vi "Performance Test 1.vi"() -> ()   [LabVIEW 2015, in "ByRef Variant Repository.lvlib"]
uses:
  ByRef Variant Repository.lvlib
  <vilib>/Analysis/1siggen.llb/Riffle Array (I32).vi
  <userlib>/_OpenG.lib/array/array.llb/Reorder 1D Array2 (String)__ogtk.vi
  <userlib>/_OpenG.lib/array/array.llb/Reorder 1D Array2 (SGL)__ogtk.vi
  <vilib>/Analysis/NI_AALBase.lvlib
panel:
  out "Data OK":bool
  out "Read Time [s]":dbl
  out "Write Time [s]":dbl
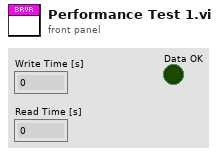
[diagram p1: front panel]
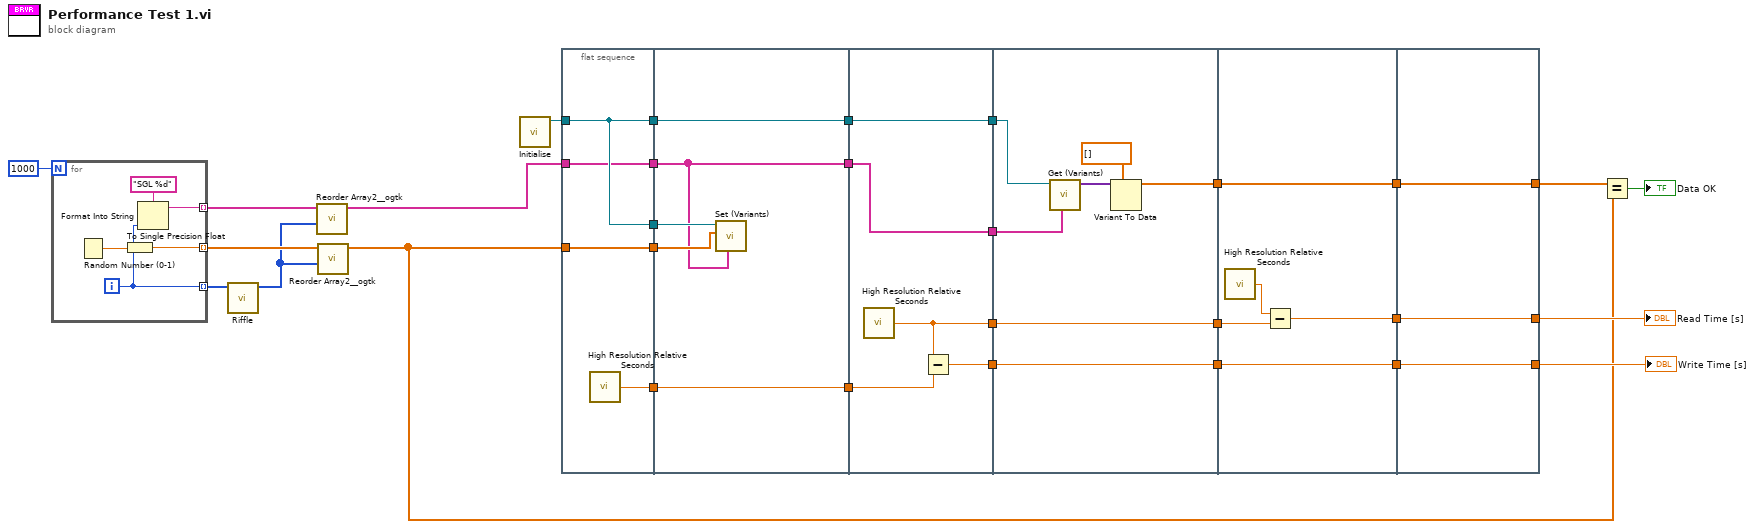
[diagram p0: block diagram]
diagram:
  n1 = for {
    N: 1000 -> [_]
    tunnel: [w34] -> w21 mode=indexing
    tunnel: [w32] -> w23 mode=indexing
    tunnel: [w31] -> w25 mode=indexing
    i -> [w31]
    n2 = Random Number (0-1)() -> (number: 0 to 1=w35:dbl)
    n3 = To Single Precision Float(number=w35) -> (single precision float=w34:sgl)
    n4 = Format Into String(format string="SGL %d", w31) -> (resulting string=w32:string)  [unwired: 2 in, 1 out]
  }
  n5 = call-poly <vilib>:"Riffle.vi"("X"=w25) -> ("Riffled {X}"=w20:i32[])  [unwired: 8 in, 2 out]
  n6 = call-poly <userlib>:"Reorder Array2__ogtk.vi"("indices"=w20, "array"=w23) -> ("reordered array"=w24:string[])  [unwired: 9 in]
  n7 = call-poly <userlib>:"Reorder Array2__ogtk.vi"("indices"=w20, "array"=w21) -> ("reordered array"=w22:sgl[])  [unwired: 9 in]
  n8 = call "Initialise.vi"() -> ("ByRef Variant Repsitory out"=w1:refnum<data-value>)  [unwired: 9 in, 1 out]
  n9 = flat-sequence {
    tunnel: w22 -> [w39]
    tunnel: w1 -> [w38]
    tunnel: [w38] -> w19
    tunnel: [w39] -> w18
    tunnel: [w38] -> w17
    tunnel: [w37] -> w16
    tunnel: w24 -> [w37]
    tunnel: [w36] -> w15
    tunnel: w19 -> [w42]
    tunnel: w18 -> [w41]
    tunnel: [w44] -> w14
    tunnel: w17 -> [w44]
    tunnel: [w40] -> w13
    tunnel: w16 -> [w40]
    tunnel: [w43] -> w12
    tunnel: w15 -> [w43]
    tunnel: [w49] -> w11
    tunnel: w14 -> [w49]
    tunnel: [w48] -> w10
    tunnel: w13 -> [w48]
    tunnel: w12 -> [w47]
    tunnel: [w46] -> w9
    tunnel: [w45] -> w8
    tunnel: w11 -> [w54]
    tunnel: w10 -> [w50]
    tunnel: [w51] -> w7
    tunnel: [w56] -> w6
    tunnel: w9 -> [w56]
    tunnel: [w55] -> w5
    tunnel: w8 -> [w55]
    tunnel: w7 -> [w61]
    tunnel: [w61] -> w4
    tunnel: w6 -> [w60]
    tunnel: [w58] -> w3
    tunnel: [w57] -> w2
    tunnel: w5 -> [w57]
    tunnel: w4 -> [w64]
    tunnel: [w64] -> w29
    tunnel: [w63] -> w27
    tunnel: w3 -> [w63]
    tunnel: [w62] -> w26
    tunnel: w2 -> [w62]
    frame #0 {
      n10 = call <vilib>:"High Resolution Relative Seconds.vi"() -> ("relative seconds"=w36:dbl)
    }
    frame #1 {
      n11 = call "Set (Variants).vi"("Tags"=w40, "Values"=w41, "ByRef Variant Repsitory in"=w42) -> ()  [unwired: 7 in, 1 out]
    }
    frame #2 {
      n12 = call <vilib>:"High Resolution Relative Seconds.vi"() -> ("relative seconds"=w46:dbl)
      n13 = Subtract(x=w46, y=w47) -> (x-y=w45:dbl)
    }
    frame #3 {
      n14 = call "Get (Variants).vi"("Tags"=w50, "ByRef Variant Repsitory in"=w54) -> ("Values"=w53:variant[])  [unwired: 7 in, 1 out]
      n15 = Variant To Data(type=sgl[] [] ("reordered array"), Variant=w53) -> (data=w51:sgl[])  [unwired: 1 in, 1 out]
    }
    frame #4 {
      n16 = call <vilib>:"High Resolution Relative Seconds.vi"() -> ("relative seconds"=w59:dbl)
      n17 = Subtract(x=w59, y=w60) -> (x-y=w58:dbl)
    }
    frame #5 {
    }
  }
  n18 = Equal?(x=w29, y=w22) -> (x = y?=→"Data OK":bool)
  "Read Time [s]" <- w27
  "Write Time [s]" <- w26
